vi "Lorentz_Fit_DLL_Test.vi"() -> ()   [LabVIEW 2020]
doc: "Test the operation of the Lorentzian Model Fit DLL inside LabVIEW\n\nThe code should do the following\n1. read in a data file containing measured LLM data [freq (MHz), spctrm (dBm)]\n1a. select a subset of the data from some subset of the freq range (optional)\n2. provide initial guesses for the fitting parameters\n3. call the function Lorentz_Fit from the DLL\n\nR. Sheehan 9 - 11 - 2021"
uses:
  <vilib>/Utility/file.llb/Read Delimited Spreadsheet (DBL).vi
panel:
  in  "Fcentre / MHz":dbl=80.0
  out "gof_stats":dbl[](array[numeric])=[4799.0, 1.000625521267723, 0.9428903903200956, 0.4850704566774246]
  out "a_pars":dbl[](array[numeric])=[2.3238013033110674, 80.0, 1.3781481716459836]
  in  "Freqs":T1={"Ffitlo / MHz"=70.0, "Fcentre / MHz"=80.0, "Ffithi / MHz"=90.0, "LLest / MHz"=2.6187499999999915, "Peak Est / nW"=0.0, "Gau stdev / MHz "=2.6187499999999915}
  out "FileName":path=path "C:/Users/robertsheehan/Programming/LabVIEW/Textronix_RSA2203A/Sample_Data/Smpl_LLM_1.txt"
  in  "Ffithi / MHz":dbl=95.0
  in  "Ffitlo / MHz":dbl=65.0
  out "Fmax / MHz":dbl=80.19375
  out "LLest / MHz":dbl=2.299999999999997
  out "Pmax / nW":dbl=1.4094510581310635e-06
  out "Pmax / dBm":dbl=-58.5095
  out "Flo / MHz":dbl=60.0
  out "Fhi / MHz":dbl=100.0
  out "LLM Output":cluster{"all rows":dbl[], "all rows":dbl[]}[](graph)
  out "TheData":dbl[][](array[numeric])
  # "Amp. Par\n\nAOM Freq / MHz\n\nLL / MHz"
  # "chi^{2} for the fit\n\nchi^{2} / nu\n\nR^{2}\n\nGOF"
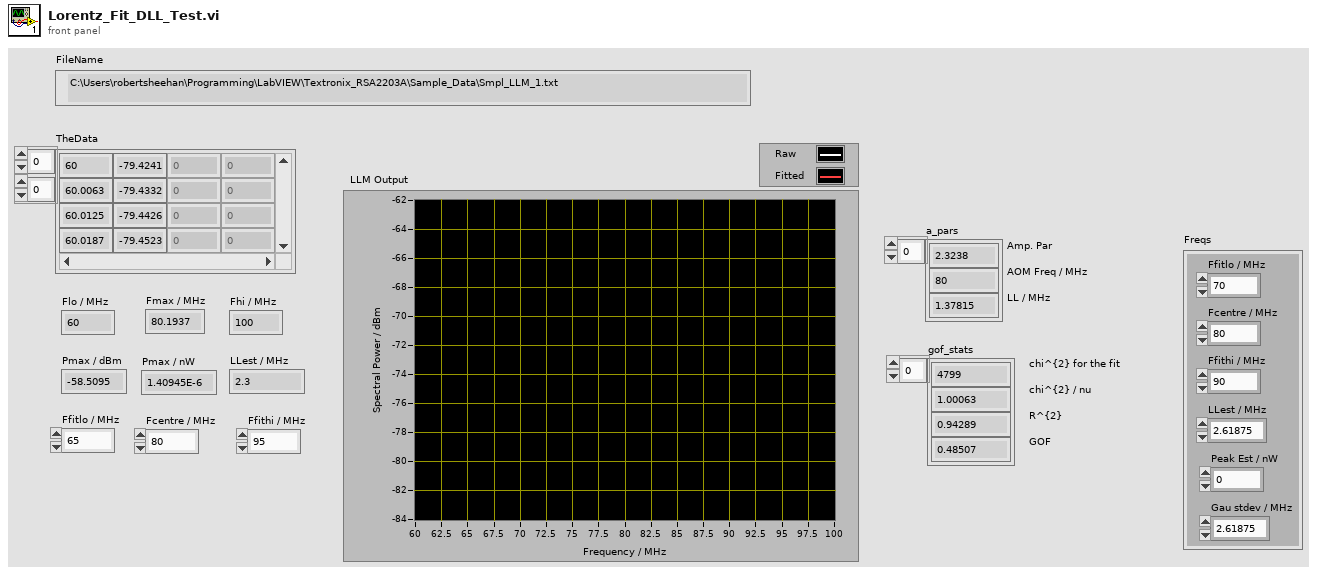
[diagram p1: front panel]
types:
  T1 = cluster{"Ffitlo / MHz":dbl, "Fcentre / MHz":dbl, "Ffithi / MHz":dbl, "LLest / MHz":dbl, "Peak Est / nW":dbl, "Gau stdev / MHz ":dbl}
  T2 = cluster{"freq_fit_data":dbl[], "spctrm_fit_data":dbl[]}
  T3 = cluster{"freq_fit_data":dbl[], "spctrm_fit_data":dbl[]}[]
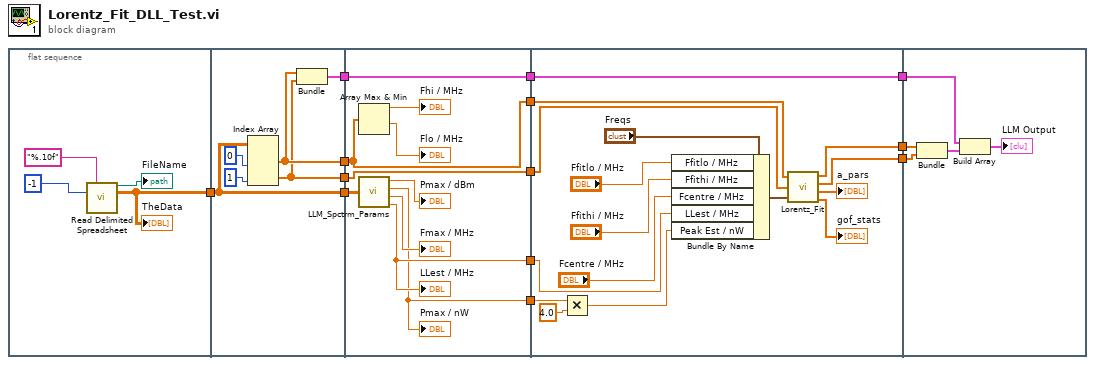
[diagram p0: block diagram]
diagram:
  n1 = flat-sequence {
    tunnel: [w15] -> w13
    tunnel: w13 -> [w21]
    tunnel: [w20] -> w12
    tunnel: [w21] -> w11
    tunnel: [w19] -> w10
    tunnel: [w18] -> w9
    tunnel: w12 -> [w26]
    tunnel: w11 -> [w32]
    tunnel: w10 -> [w25]
    tunnel: w9 -> [w27]
    tunnel: [w28] -> w8
    tunnel: [w27] -> w6
    tunnel: [w26] -> w3
    tunnel: [w25] -> w2
    tunnel: [w24] -> w1
    tunnel: w8 -> [w43]
    tunnel: [w42] -> w7
    tunnel: w6 -> [w42]
    tunnel: [w41] -> w5
    tunnel: [w40] -> w4
    tunnel: w3 -> [w39]
    tunnel: w2 -> [w38]
    tunnel: w1 -> [w36]
    tunnel: w7 -> [w54]
    tunnel: w5 -> [w53]
    tunnel: w4 -> [w52]
    frame #0 {
      n2 = call-poly <vilib>:"Read Delimited Spreadsheet.vi"("format (%.3f)"="%.10f", "number of rows (all:-1)"=-1) -> ("new file path (Not A Path if cancelled)"=→"FileName":path, "all rows"=w15:dbl[][])  [unwired: 8 in, 4 out]
      "TheData" <- w15
    }
    frame #1 {
      n3 = Index Array(array=w21, index (col) #1=0 ("disabled index (col)"), index (col) #2=1 ("index (col)")) -> (element #1=w20:dbl[], element #2=w19:dbl[])  [unwired: 2 in]
      n4 = Bundle("all rows"=w20, "all rows"=w19) -> (w18:cluster{"all rows":dbl[], "all rows":dbl[]})  [unwired: 1 in]
    }
    frame #2 {
      n5 = Array Max & Min(array=w26) -> (max value=→"Fhi / MHz":dbl, min value=→"Flo / MHz":dbl)  [unwired: 2 out]
      n6 = call "LLM_Spctrm_Params.vi"("Data"=w32) -> ("Pmax / dBm"=→"Pmax / dBm":dbl, "Pmax / nW"=w24:dbl, "Fmax / MHz"=→"Fmax / MHz":dbl, "LL / MHz"=w28:dbl)
      "Pmax / nW" <- w24
      "LLest / MHz" <- w28
    }
    frame #3 {
      n7 = Multiply(x=w36, y=4.0) -> (x*y=w34:dbl)
      n8 = Bundle By Name(cluster="Freqs", "Ffitlo / MHz"="Ffitlo / MHz", "Ffithi / MHz"="Ffithi / MHz", "Fcentre / MHz"="Fcentre / MHz", "LLest / MHz"=w43, "Peak Est / nW"=w34) -> (w48:T1)
      n9 = call "Lorentz_Fit.vi"("Freq_Data"=w39, "Scptrm_Data"=w38, "Freqs"=w48) -> ("freq_fit_data"=w41:dbl[], "spctrm_fit_data"=w40:dbl[], "a_pars"=→"a_pars":dbl[], "gof_stats"=→"gof_stats":dbl[])
    }
    frame #4 {
      n10 = Bundle("freq_fit_data"=w53, "spctrm_fit_data"=w52) -> (w51:T2)  [unwired: 1 in]
      n11 = Build Array(w54, w51) -> (→"LLM Output":T3)
    }
  }
